vi "Add Scheduled Message to Minor Frame.vi"(8 "error in":errorcluster, 9 "Scheduled Message Config in":T1[](array[typedef]), 11 "MinorFrame in":refnum<k24>) -> (0 "error out":errorcluster, 3 "MinorFrame out":refnum<k24>)   [LabVIEW 2020, in "Ballard_1553_Hardware_ni.lvlib"]
uses:
  Ballard_1553_Hardware_ni.lvlib
  C:/Users/Administrator/Desktop/GIT/Ballard-MIL-STD-1553-Custom-Device/Source/System Explorer/SubVIs/Parse XML Ballard/1.2/BTIXML_SerDes.dll
  Ballard-MIL-STD-1553-Custom-Device/Source/System Explorer/SubVIs/Parse XML Ballard/1.2/BTIXML_SerDes.dll
  _typedefs/schedItem1553_type.ctl
  _typedefs/frame_entry_type.ctl
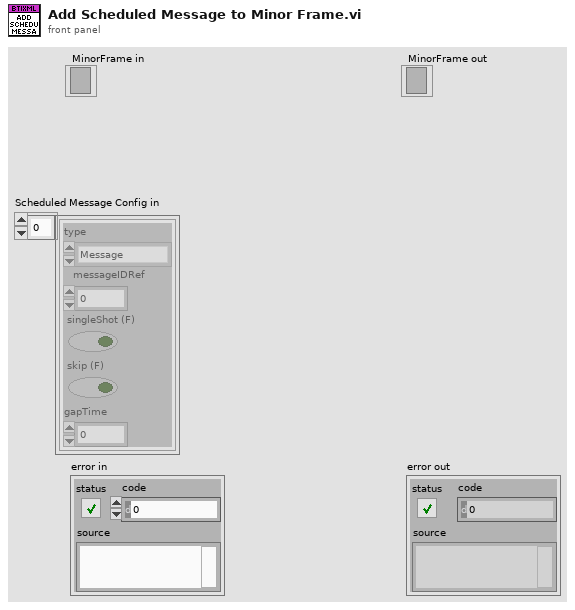
[diagram p1: front panel]
types:
  T1 = typedef "Ballard_1553_Hardware_ni.lvlib/schedItem1553_type.ctl" = cluster{"type":T2, "messageIDRef":i32, "singleShot (F)":bool, "skip (F)":bool, "gapTime":dbl}
  T2 = typedef "Ballard_1553_Hardware_ni.lvlib/frame_entry_type.ctl" = enum16{"Message", "Gap", "Pulse", "Log", "Pause", "Restart", "Halt"}
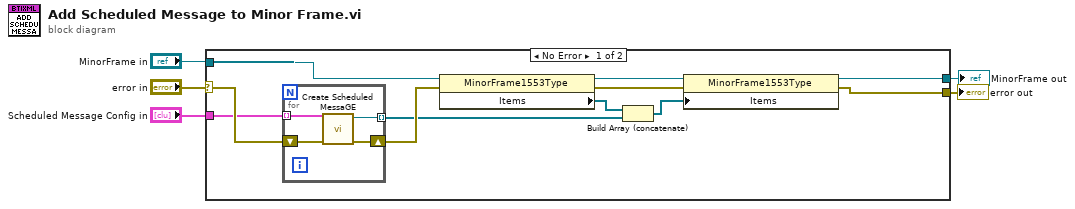
[diagram p0: block diagram]
diagram:
  n1 = case shown="No Error" "error in" {
    selector: "error in" -> [w10 w21]
    tunnel: [w13 w21] -> w5
    tunnel: [w14 w22] -> w4
    tunnel: "MinorFrame in" -> [w16 w22]
    tunnel: "Scheduled Message Config in" -> [w9 _]
    frame No Error {
      n2 = for {
        shift-right: [w18] -> w8
        shift-left: w10 -> [w20]
        tunnel: w9 -> [w19] mode=indexing
        tunnel: [w17] -> w7 mode=indexing
        n3 = call "Create Scheduled MessaGE.vi"("error in"=w20, "1553 Scheduled Message Configuration in"=w19) -> ("error out"=w18:errorcluster, "message out"=w17:refnum<k24>)  [unwired: 8 in]
      }
      n4 = property class="MinorFrame1553Type"(reference=w16, error in=w8) -> (reference out=w15:refnum<k24>, error out=w12:errorcluster, "Items"=w11:refnum<k24>[])
      n5 = Build Array (concatenate)(w11, w7) -> (w6:refnum<k24>[])
      n6 = property class="MinorFrame1553Type"(reference=w15, error in=w12, "Items"=w6) -> (reference out=w14:refnum<k24>, error out=w13:errorcluster)
    }
    frame Error {
    }
  }
  "error out" <- w5
  "MinorFrame out" <- w4
